vi "example.vi"() -> ()   [LabVIEW 2013]
uses:
  <vilib>/Analysis/baseanly.llb/A x Vector.vi
  <vilib>/Analysis/NI_AALBase.lvlib
panel:
  out "A x B":dbl[](array[numeric]) format="%.2f"
  in  "B":dbl[](array[numeric])
  in  "A":dbl[][](array[numeric])
  out "concatenated string":string
  in  "s":string
  out "x+y":dbl
  in  "y":dbl
  in  "x":dbl
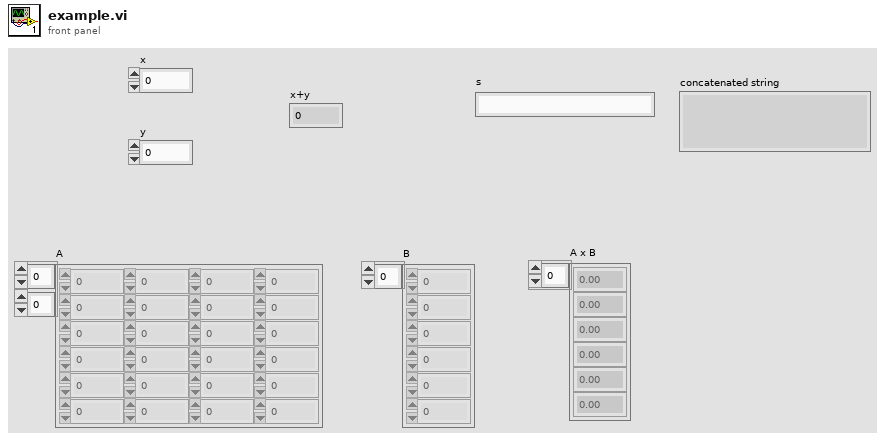
[diagram p1: front panel]
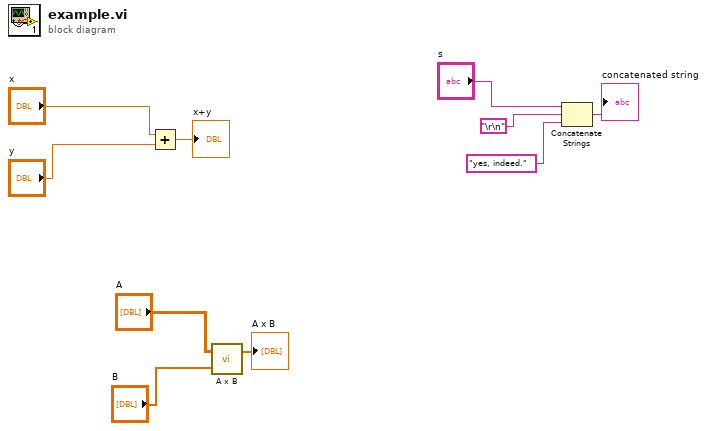
[diagram p0: block diagram]
diagram:
  n1 = Add(x="x", y="y") -> (x+y=→"x+y":dbl)
  n2 = call-poly <vilib>:"A x B.vi"("Vector"="B", "A"="A") -> ("A x Vector"=→"A x B":dbl[])  [unwired: 1 out]
  n3 = Concatenate Strings("s", "\r\n", "yes, indeed." ("string")) -> (→"concatenated string":string)
